vi "newsubvi Robot Get Z.vi"(0 "VISA In":refnum<visa-resource-name>) -> (1 "VISA Out":refnum<visa-resource-name>, 2 "ZPosition":i32, 3 "error out":errorcluster)   [LabVIEW 2012]
doc: "Returns Absloute value of Z Position"
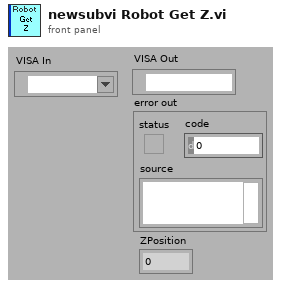
[diagram p1: front panel]
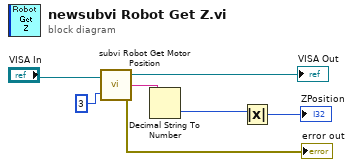
[diagram p0: block diagram]
diagram:
  n1 = call "subvi Robot Get Motor Position.vi"("VISA In"="VISA In", "Motor Number"=3) -> ("VISA Out"=→"VISA Out":refnum<visa-resource-name>, "Motor Position"=w2:string, "error out"=→"error out":errorcluster)  [unwired: 1 out]
  n2 = Decimal String To Number(string=w2) -> (number=w1:i32)  [unwired: 3 out]
  n3 = Absolute Value(x=w1) -> (abs(x)=→"ZPosition":i32)
